vi "Caller.vi"(9 "Priority?":bool, 10 "Msg":refnum<class "Msg.lvclass">, 11 "Ex Queue Actor in":refnum<class "Ex Queue Actor.lvclass">) -> (3 "Ex Queue Actor out":refnum<class "Ex Queue Actor.lvclass">)   [LabVIEW 2021, in "Ex Queue Actor.lvlib" / "Ex Queue Actor.lvclass"]
uses:
  Ex Queue Actor.lvclass
  Actor/Msg/Msg.lvclass
  Ex Queue Actor.lvclass/Ex Queue Actor.ctl
  Actor/Queue Actor/Queue Actor.lvclass
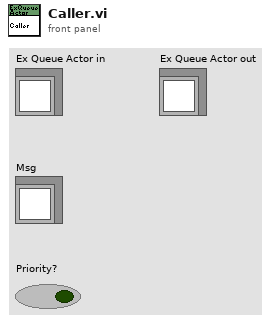
[diagram p1: front panel]
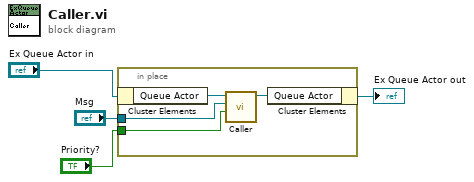
[diagram p0: block diagram]
diagram:
  n1 = in-place {
    in-place-border: "Priority?" -> [w8]
    in-place-border: "Msg" -> [w7]
    n2 = in-place-cluster #1("Ex Queue Actor in") -> ("Queue Actor"=w6:refnum<class "Queue Actor.lvclass">)
    n3 = call-dynamic "Caller.vi"("Priority?"=w8, "Msg"=w7, "Queue Actor in"=w6) -> ("Queue Actor out"=w5:refnum<class "Queue Actor.lvclass">)  [unwired: 8 in]
    n4 = in-place-cluster #1("Queue Actor"=w5) -> (→"Ex Queue Actor out":refnum<class "Ex Queue Actor.lvclass">)
  }
